vi "escape_special_characters.vi"(1 "String in":string) -> (0 "String out":string)   [LabVIEW 2010]
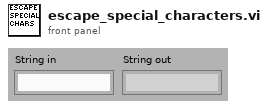
[diagram p1: front panel]
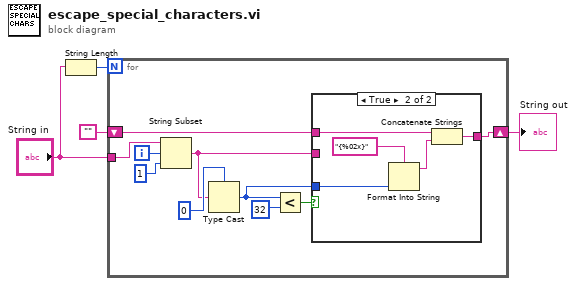
[diagram p0: block diagram]
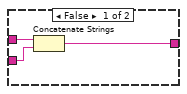
[diagram p2: hidden frame]
diagram:
  n1 = String Length(string="String in") -> (length=w4:i32)
  n2 = for {
    N: w4 -> [_]
    tunnel: "String in" -> [w12]
    shift-right: [w6] -> w1
    shift-left: "" -> [w8]
    i -> [w13]
    n3 = String Subset(string=w12, offset (0)=w13, length (rest)=1 ("length (rest)")) -> (substring=w5:string)
    n4 = Type Cast(type=u8 0, x=w5) -> (*(type *) &x=w7:u8)
    n5 = Less?(x=w7, y=u8 32) -> (x < y?=w9:bool)
    n6 = case shown="True" w9 {
      tunnel: w8 -> [w17 w22]
      tunnel: w7 -> [_ w21]
      tunnel: [w15 w18] -> w6
      tunnel: w5 -> [w16 _]
      frame False {
        n7 = Concatenate Strings(w17, w16) -> (w15:string)
      }
      frame True {
        n8 = Format Into String(format string="{%02x}", w21) -> (resulting string=w19:string)  [unwired: 2 in, 1 out]
        n9 = Concatenate Strings(w22, w19) -> (w18:string)
      }
    }
  }
  "String out" <- w1
